vi "Write Generator Data to Optimization.vi"(7 "Bus by ID":T1[](array[typedef]), 8 "error in":errorcluster, 11 "Generic Optimization in":refnum<class "Generic Optimization.lvclass">) -> (0 "error out":errorcluster, 3 "Generic Optimization out":refnum<class "Generic Optimization.lvclass">)   [LabVIEW 2018, in "Generic Optimization Actor.lvlib" / "Generic Optimization.lvclass"]
uses:
  Generic Optimization.lvclass
  C:/Users/Administrator/Desktop/2018LabVIEW EMS/EMS Generic Actor/EMS Generic/EMS Generic.lvclass
  Optimization Controls/Bus by ID.ctl
  <vilib>/ORNL/CSEISMIC DDS/CSEISMIC DDS Base/Data Types/Controls/DeviceID.ctl
  EMS Generic Actor/EMS Generic/EMS Generic.lvclass/EMS Generic.ctl
  <vilib>/ORNL/CSEISMIC DDS/CSEISMIC DDS Base/Data Types/Generator_Info.ctl
  <vilib>/ORNL/CSEISMIC DDS/CSEISMIC DDS Base/Data Types/Controls/EfficiencyCurve.ctl
  <vilib>/ORNL/CSEISMIC DDS/CSEISMIC DDS Base/Data Types/DER_Info.ctl
  <vilib>/ORNL/CSEISMIC DDS/CSEISMIC DDS Base/CSEISMIC DDS.lvclass
  EMS Generic Actor/EMS Generic/EMS Generic.lvclass
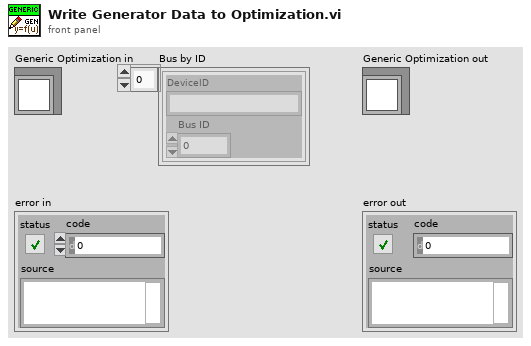
[diagram p1: front panel]
types:
  T1 = typedef "Generic Optimization Actor.lvlib/Generic Optimization.lvclass/Bus by ID.ctl" = cluster{"DeviceID":T2, "Bus ID":dbl}
  T2 = typedef "CSEISMIC DDS.lvlib/CSEISMIC DDS.lvclass/DeviceID.ctl" = string
  T3 = typedef "CSEISMIC DDS.lvlib/CSEISMIC DDS.lvclass/DER_Info.ctl" = cluster{"DeviceID":T2, "LineConfig":u8[], "NominalVoltage(V)":dbl, "PowerRating(kVA)":dbl, "VFControl":bool, "PControl":bool, "QControl":bool, "PFControl":bool, "PVControl":bool, "Droop":bool, "DroopConfigurable":bool, "Unbalanced":bool}
  T4 = typedef "CSEISMIC DDS.lvlib/CSEISMIC DDS.lvclass/Generator_Info.ctl" = cluster{"DeviceID":T2, "Voltage (V)":dbl, "MinimumPower (kVA)":dbl, "EnergyRating (kWh)":dbl, "RampRate (kW/s)":dbl, "MaxPowerFactorLeading":dbl, "MaxPowerFactorLagging":dbl, "EfficiencyCurve":T5, "StartCost":dbl, "FuelCost":dbl, "StartTime (s)":dbl}
  T5 = typedef "CSEISMIC DDS.lvlib/CSEISMIC DDS.lvclass/EfficiencyCurve.ctl" = cluster{"Power (kW)":dbl[], "Efficiency (%)":dbl[]}
  T6 = typedef "EMS Generic Actor.lvlib/EMS Generic.lvclass/Data Type DVRs.ctl" = cluster{"IED_Status":refnum<data-value>, "IED_Status_0":refnum<data-value>, "DER_Measurement":refnum<data-value>, "DER_Info":refnum<data-value>, "DER_Status":refnum<data-value>, "ES_Measurement":refnum<data-value>, "ES_Info":refnum<data-value>, "PV_Info":refnum<data-value>, "SmartRelay_Info":refnum<data-value>, "SmartRelay_Measurement":refnum<data-value>, "Meter_Info":refnum<data-value>, "Meter_Measurement":refnum<data-value>, "HVAC_Status":refnum<data-value>, "HVAC_Measurement":refnum<data-value>, "PriceData_RealTime":refnum<data-value>, "PriceData_Demand":refnum<data-value>, "PriceData_Energy":refnum<data-value>, "ForecastData_Long":refnum<data-value>, "ForecastData_Short":refnum<data-value>, "DER_Control":refnum<data-value>, "DER_SetPointF":refnum<data-value>, "DER_SetPointP":refnum<data-value>, "DER_SetPointQ":refnum<data-value>, "DER_SetPointPF":refnum<data-value>, "DER_SetPointV":refnum<data-value>, "PV_setCurtailment":refnum<data-value>, "PV_setRampRate":refnum<data-value>, "Relay_Control":refnum<data-value>, "Load_Control":refnum<data-value>, "HVAC_Control":refnum<data-value>, "Generator_Info":refnum<data-value>, "ForecastData_Long_Backup":refnum<data-value>, "PriceData_RealTime_Backup":refnum<data-value>}
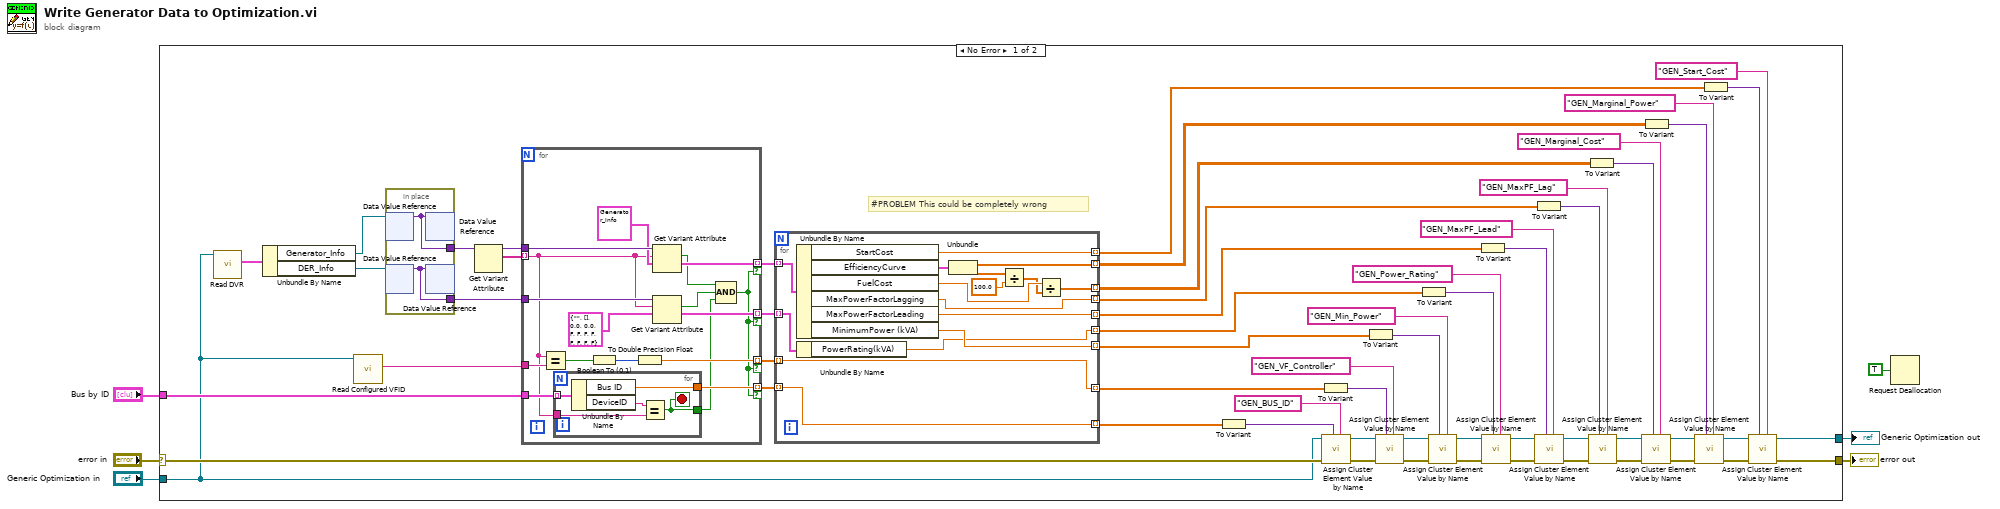
[diagram p0: block diagram]
diagram:
  n1 = case shown="No Error" "error in" {
    selector: "error in" -> [w33 w107]
    tunnel: [w60 w107] -> w6
    tunnel: "Bus by ID" -> [w18 _]
    tunnel: "Generic Optimization in" -> [w8 w108]
    tunnel: [w7 w108] -> w2
    frame No Error {
      # "#PROBLEM This could be completely wrong"
      n2 = call "Read DVR.vi"("EMS Generic in"=w8) -> ("DVR"=w23:T6)  [unwired: 9 in, 1 out]
      n3 = Unbundle By Name(w23) -> ("Generator_Info"=w22:refnum<data-value>, "DER_Info"=w12:refnum<data-value>)
      n4 = call "Read Configured VFID.vi"("EMS Generic in"=w8) -> ("VFID"=w9:T2)  [unwired: 8 in, 2 out]
      n5 = in-place {
        in-place-border: [w106] -> w21
        in-place-border: [w105] -> w11
        n6 = in-place-dvr #1(w22) -> (w106:variant)  [unwired: 1 out]
        n7 = in-place-dvr #2(w12) -> (w105:variant)  [unwired: 1 out]
        n8 = in-place-dvr #1(w106) -> ()  [unwired: 2 out]
        n9 = in-place-dvr #2(w105) -> ()  [unwired: 2 out]
      }
      n10 = Get Variant Attribute(Variant=w21) -> (duplicate Variant=w20:variant, names=w19:string[])  [unwired: 3 in, 2 out]
      n11 = for {
        tunnel: w19 -> [w89] mode=indexing
        tunnel: w20 -> [w99]
        tunnel: w9 -> [w98]
        tunnel: w18 -> [w97]
        tunnel: [w94] -> w16 mode=indexing if=w83
        tunnel: [w93] -> w15 mode=indexing if=w83
        tunnel: [w91] -> w17 mode=indexing if=w83
        tunnel: w11 -> [w90]
        tunnel: [w87] -> w10 mode=indexing if=w83
        n12 = Equal?(x=w89, y=w98) -> (x = y?=w95:bool)
        n13 = for {
          tunnel: w97 -> [w104] mode=indexing
          tunnel: w89 -> [w103]
          tunnel: [w101] -> w91
          tunnel: [w100] -> w84
          stop <- w100 stop-if-true
          n14 = Unbundle By Name(w104) -> ("Bus ID"=w101:dbl, "DeviceID"=w102:T2)
          n15 = Equal?(x=w102, y=w103) -> (x = y?=w100:bool)
        }
        n16 = Boolean To (0,1)(Boolean=w95) -> (0, 1=w96:i16)
        n17 = To Double Precision Float(number=w96) -> (double precision float=w94:dbl)
        n18 = Get Variant Attribute(Variant=w99, name=w89, default value (empty Variant)=T4 {"DeviceID"="", "Voltage (V)"=0.0, "MinimumPower (kVA)"=0.0, "EnergyRating (kWh)"=0.0, "RampRate (kW/s)"=0.0, "MaxPowerFactorLeading"=0.0, "MaxPowerFactorLagging"=0.0, "EfficiencyCurve"={"Power (kW)"=[], "Efficiency (%)"=[]}, "StartCost"=0.0, "FuelCost"=0.0, "StartTime (s)"=0.0} ("Generator_Info")) -> (found=w86:bool, value=w93:T4)  [unwired: 1 in, 2 out]
        n19 = Get Variant Attribute(Variant=w90, name=w89, default value (empty Variant)=T3 {"DeviceID"="", "LineConfig"=[], "NominalVoltage(V)"=0.0, "PowerRating(kVA)"=0.0, "VFControl"=FALSE, "PControl"=FALSE, "QControl"=FALSE, "PFControl"=FALSE, "PVControl"=FALSE, "Droop"=FALSE, "DroopConfigurable"=FALSE, "Unbalanced"=FALSE} ("DER_Info")) -> (found=w85:bool, value=w87:T3)  [unwired: 1 in, 2 out]
        n20 = Compound Arithmetic op=AND(w86, w85, w84) -> (w83:bool)
      }
      n21 = for {
        tunnel: [w77] -> w24 mode=indexing
        tunnel: [w78] -> w30 mode=indexing
        tunnel: [w82] -> w29 mode=indexing
        tunnel: [w72] -> w28 mode=indexing
        tunnel: [w81] -> w27 mode=indexing
        tunnel: [w80] -> w26 mode=indexing
        tunnel: [w79] -> w25 mode=indexing
        tunnel: w17 -> [w77] mode=indexing
        tunnel: w16 -> [w78] mode=indexing
        tunnel: w15 -> [w76] mode=indexing
        tunnel: [w74] -> w14 mode=indexing
        tunnel: [w67] -> w13 mode=indexing
        tunnel: w10 -> [w73] mode=indexing
        n22 = Unbundle By Name(w76) -> ("StartCost"=w79:dbl, "EfficiencyCurve"=w75:T5, "FuelCost"=w69:dbl, "MaxPowerFactorLagging"=w80:dbl, "MaxPowerFactorLeading"=w81:dbl, "MinimumPower (kVA)"=w82:dbl)
        n23 = Unbundle By Name(w73) -> ("PowerRating(kVA)"=w72:dbl)
        n24 = Unbundle(w75) -> ("Power (kW)"=w74:dbl[], "Efficiency (%)"=w70:dbl[])
        n25 = Divide(x=w70, y=100.0) -> (x/y=w68:dbl[])
        n26 = Divide(x=w69, y=w68) -> (x/y=w67:dbl[])
      }
      n27 = To Variant(anything=w24) -> (Variant=w31:variant)
      n28 = To Variant(anything=w30) -> (Variant=w61:variant)
      n29 = call "Assign Cluster Element Value by Name.vi"("Element Name"="GEN_BUS_ID" ("Keyword Name"), "Value"=w31, "error in"=w33, "Generic Optimization"=w8) -> ("error out"=w63:errorcluster, "Generic Optimization out"=w64:refnum<class "Generic Optimization.lvclass">)  [unwired: 6 in]
      n30 = To Variant(anything=w29) -> (Variant=w34:variant)
      n31 = call "Assign Cluster Element Value by Name.vi"("Element Name"="GEN_VF_Controller" ("Keyword Name"), "Value"=w61, "error in"=w63, "Generic Optimization"=w64) -> ("error out"=w65:errorcluster, "Generic Optimization out"=w66:refnum<class "Generic Optimization.lvclass">)  [unwired: 6 in]
      n32 = To Variant(anything=w28) -> (Variant=w36:variant)
      n33 = call "Assign Cluster Element Value by Name.vi"("Element Name"="GEN_Min_Power" ("Keyword Name"), "Value"=w34, "error in"=w65, "Generic Optimization"=w66) -> ("error out"=w49:errorcluster, "Generic Optimization out"=w48:refnum<class "Generic Optimization.lvclass">)  [unwired: 6 in]
      n34 = To Variant(anything=w27) -> (Variant=w38:variant)
      n35 = call "Assign Cluster Element Value by Name.vi"("Element Name"="GEN_Power_Rating" ("Keyword Name"), "Value"=w36, "error in"=w49, "Generic Optimization"=w48) -> ("error out"=w50:errorcluster, "Generic Optimization out"=w47:refnum<class "Generic Optimization.lvclass">)  [unwired: 6 in]
      n36 = To Variant(anything=w26) -> (Variant=w40:variant)
      n37 = call "Assign Cluster Element Value by Name.vi"("Element Name"="GEN_MaxPF_Lead" ("Keyword Name"), "Value"=w38, "error in"=w50, "Generic Optimization"=w47) -> ("error out"=w51:errorcluster, "Generic Optimization out"=w46:refnum<class "Generic Optimization.lvclass">)  [unwired: 6 in]
      n38 = To Variant(anything=w13) -> (Variant=w54:variant)
      n39 = call "Assign Cluster Element Value by Name.vi"("Element Name"="GEN_MaxPF_Lag" ("Keyword Name"), "Value"=w40, "error in"=w51, "Generic Optimization"=w46) -> ("error out"=w52:errorcluster, "Generic Optimization out"=w45:refnum<class "Generic Optimization.lvclass">)  [unwired: 6 in]
      n40 = call "Assign Cluster Element Value by Name.vi"("Element Name"="GEN_Marginal_Cost" ("Keyword Name"), "Value"=w54, "error in"=w52, "Generic Optimization"=w45) -> ("error out"=w57:errorcluster, "Generic Optimization out"=w56:refnum<class "Generic Optimization.lvclass">)  [unwired: 6 in]
      n41 = To Variant(anything=w14) -> (Variant=w58:variant)
      n42 = call "Assign Cluster Element Value by Name.vi"("Element Name"="GEN_Marginal_Power" ("Keyword Name"), "Value"=w58, "error in"=w57, "Generic Optimization"=w56) -> ("error out"=w53:errorcluster, "Generic Optimization out"=w44:refnum<class "Generic Optimization.lvclass">)  [unwired: 6 in]
      n43 = To Variant(anything=w25) -> (Variant=w42:variant)
      n44 = call "Assign Cluster Element Value by Name.vi"("Element Name"="GEN_Start_Cost" ("Keyword Name"), "Value"=w42, "error in"=w53, "Generic Optimization"=w44) -> ("error out"=w60:errorcluster, "Generic Optimization out"=w7:refnum<class "Generic Optimization.lvclass">)  [unwired: 6 in]
    }
    frame Error {
    }
  }
  "error out" <- w6
  "Generic Optimization out" <- w2
  n45 = Request Deallocation(TRUE ("flag")) -> ()
